vi "Boolean Reference.vi"(8 "error in":errorcluster, 10 "Value":bool, 11 "Boolean in":refnum<vi>) -> (0 "error out":errorcluster)   [LabVIEW 2018]
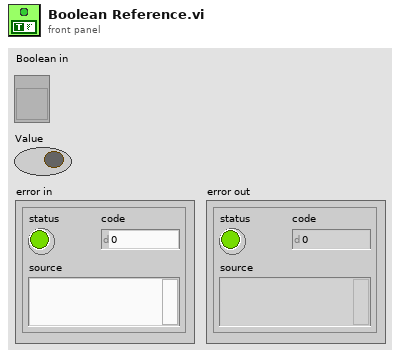
[diagram p1: front panel]
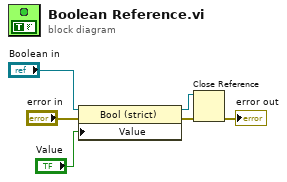
[diagram p0: block diagram]
diagram:
  n1 = property class="Bool (strict)"(reference="Boolean in", error in="error in", "Value"="Value") -> (reference out=w5:refnum<vi>, error out=w6:errorcluster)
  n2 = Close Reference(reference=w5, error in (no error)=w6) -> (error out=→"error out":errorcluster)
